vi "set window title version.vi"(11 "userInterface":T1) -> ()   [LabVIEW 2018]
uses:
  type defs/UI loop data.ctl
types:
  T1 = typedef "UI loop data.ctl" = cluster{"params":cluster{"channelConfigPath":path, "version":string}, "vars":cluster{"tempOffsets":dbl[], "encoderFallingEdge":bool, "controlRefs":cluster{"mainVI":refnum<vi>, "menu":refnum<k9>, "motorStart":refnum<vi>, "butterfly":refnum<vi>, "ball":refnum<vi>, "speed":refnum<vi>, "logLimit":refnum<vi>, "pointLimit":refnum<vi>, "logData":refnum<vi>}}}
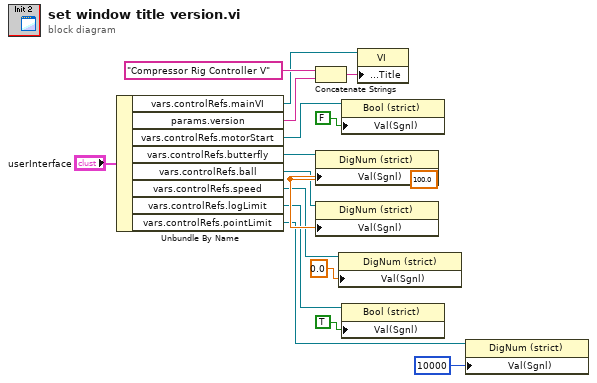
[diagram p0: block diagram]
diagram:
  w9 = 100.0 ("targetSpeed")
  n1 = Unbundle By Name("userInterface") -> ("vars.controlRefs.mainVI"=w12:refnum<vi>, "params.version"=w15:string, "vars.controlRefs.motorStart"=w6:refnum<vi>, "vars.controlRefs.butterfly"=w5:refnum<vi>, "vars.controlRefs.ball"=w4:refnum<vi>, "vars.controlRefs.speed"=w3:refnum<vi>, "vars.controlRefs.logLimit"=w2:refnum<vi>, "vars.controlRefs.pointLimit"=w1:refnum<vi>)
  n2 = Concatenate Strings("Compressor Rig Controller V" ("string"), w15) -> (w14:string)
  n3 = property on="Property Node" class="DigNum (strict)"(reference=w5, "Val(Sgnl)"=w9) -> ()  [unwired: 1 in, 2 out]
  n4 = property on="Property Node" class="DigNum (strict)"(reference=w4, "Val(Sgnl)"=w9) -> ()  [unwired: 1 in, 2 out]
  n5 = property on="Property Node" class="DigNum (strict)"(reference=w3, "Val(Sgnl)"=0.0 ("targetSpeed")) -> ()  [unwired: 1 in, 2 out]
  n6 = property on="Property Node" class="Bool (strict)"(reference=w6, "Val(Sgnl)"=FALSE ("Value (Signaling)")) -> ()  [unwired: 1 in, 2 out]
  n7 = property on="Property Node" class="Bool (strict)"(reference=w2, "Val(Sgnl)"=TRUE ("Value (Signaling)")) -> ()  [unwired: 1 in, 2 out]
  n8 = property class="VI"(reference=w12, "Front Panel.Title"=w14) -> ()  [unwired: 1 in, 2 out]
  n9 = property on="Property Node" class="DigNum (strict)"(reference=w1, "Val(Sgnl)"=u32 10000 ("Value (Signaling)")) -> ()  [unwired: 1 in, 2 out]
